vi "Initialise Hardware Splash 2.0.vi"(8 "error in (no error)":errorcluster) -> (0 "error out":errorcluster, 2 "VISA Refnum out":refnum<visa-resource-name>, 3 "Enabled Hardware out":T1={"Confocal"={"Enable"=TRUE, "Status"=FALSE, "Device"="Confocal"}, "Pinhole"={"Enable"=TRUE, "Status"=FALSE, "Device"="Pinhole"}, "PIFOC"={"Enable"=TRUE, "Status"=FALSE, "Device"="Piezo"}, "iFlex"={"Enable"=TRUE, "Status"=FALSE, "Device"="iFlex"}, "Manlight"={"Enable"=TRUE, "Status"=FALSE, "Device"="Manlight"}, "SLM"={"Enable"=TRUE, "Status"=FALSE, "Device"="SLM"}, "Camera"={"Enable"=FALSE, "Status"=FALSE, "Device"="Camera"}})   [LabVIEW 2020]
uses:
  _Controls/Enabled Hardware.ctl
panel:
  out "All Enabled and connected":bool
  in  "Enabled Hardware":T1={"Confocal"={"Enable"=TRUE, "Status"=FALSE, "Device"="Confocal"}, "Pinhole"={"Enable"=TRUE, "Status"=FALSE, "Device"="Pinhole"}, "PIFOC"={"Enable"=TRUE, "Status"=FALSE, "Device"="Piezo"}, "iFlex"={"Enable"=TRUE, "Status"=FALSE, "Device"="iFlex"}, "Manlight"={"Enable"=TRUE, "Status"=FALSE, "Device"="Manlight"}, "SLM"={"Enable"=TRUE, "Status"=FALSE, "Device"="SLM"}, "Camera"={"Enable"=FALSE, "Status"=FALSE, "Device"="Camera"}}
  in  "Review":bool
  in  "Scan For Missing":bool
  in  "animation":u16(ring)
  out "Status":string
  in  "Start":bool
  # "TweezerTron"
  # "Scanning for system hardware."
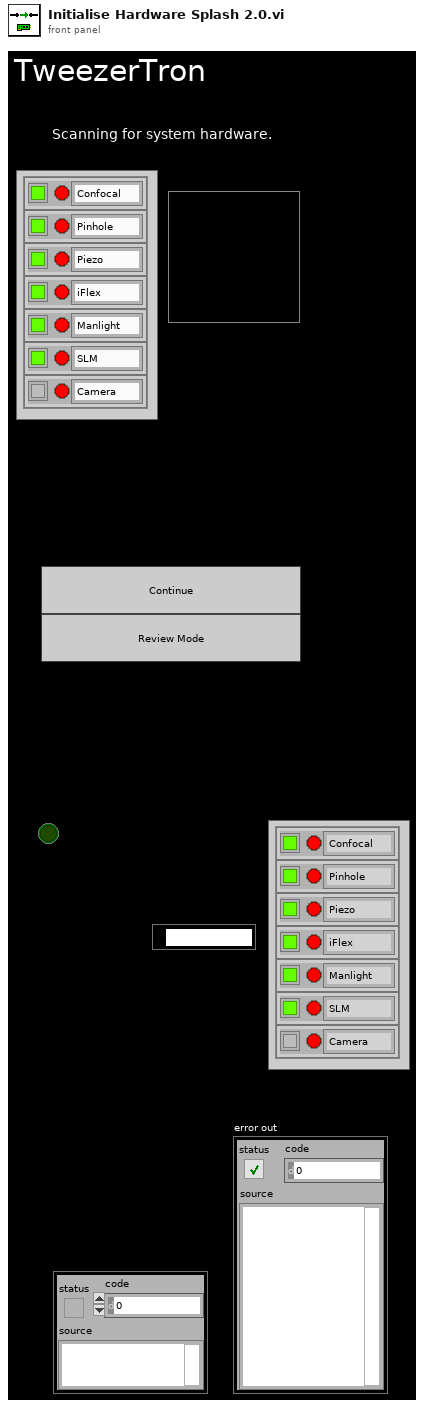
[diagram p1: front panel]
types:
  T1 = typedef "Enabled Hardware.ctl" = cluster{"Confocal":cluster{"Enable":bool, "Status":bool, "Device":string}, "Pinhole":cluster{"Enable":bool, "Status":bool, "Device":string}, "PIFOC":cluster{"Enable":bool, "Status":bool, "Device":string}, "iFlex":cluster{"Enable":bool, "Status":bool, "Device":string}, "Manlight":cluster{"Enable":bool, "Status":bool, "Device":string}, "SLM":cluster{"Enable":bool, "Status":bool, "Device":string}, "Camera":cluster{"Enable":bool, "Status":bool, "Device":string}}
  T2 = cluster{"Enable":bool, "Status":bool, "Device":string}
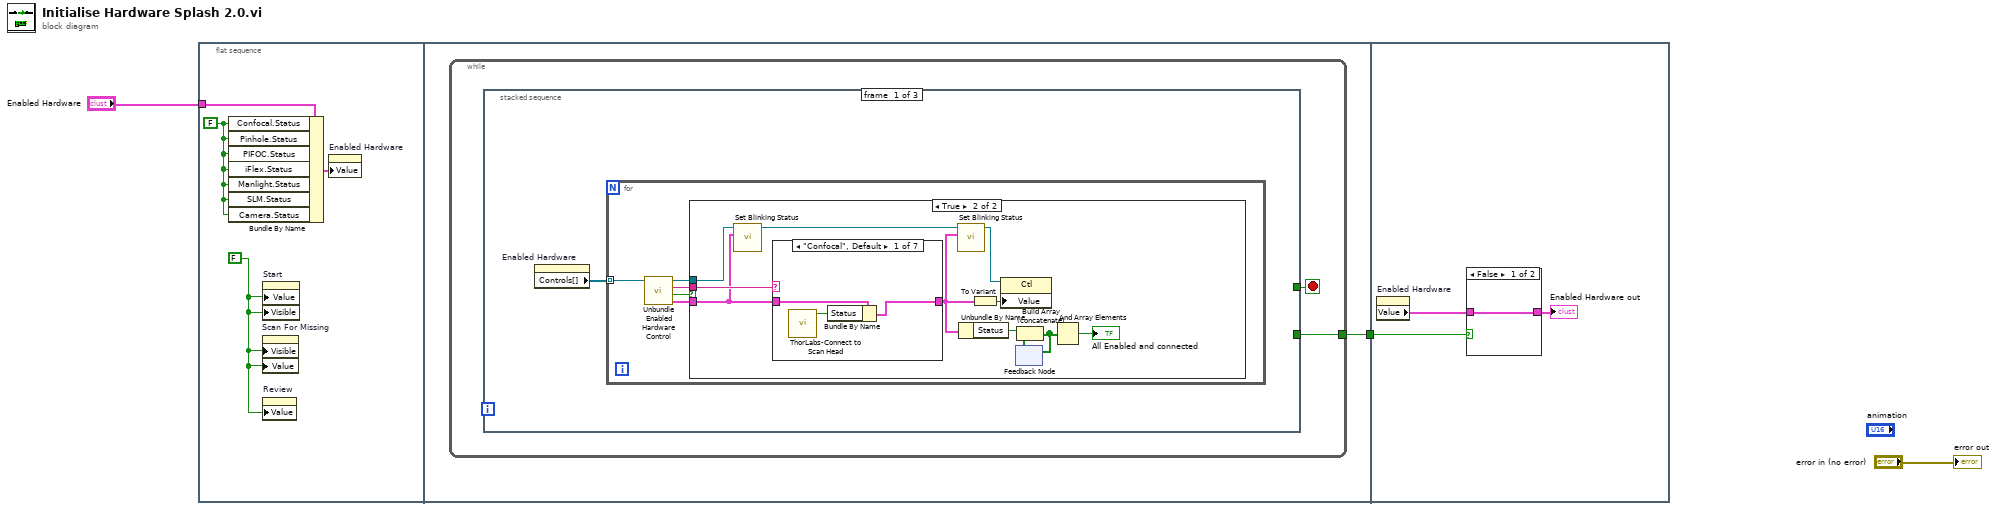
[diagram p0: block diagram]
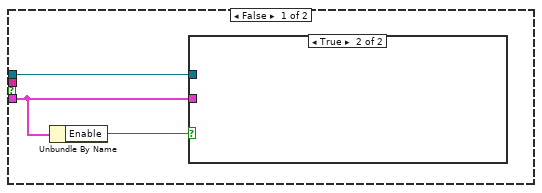
[diagram p2: hidden frame]
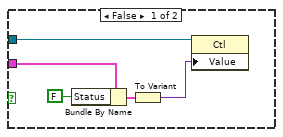
[diagram p3: hidden frame]
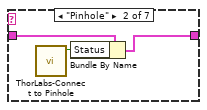
[diagram p4: hidden frame]
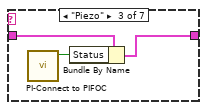
[diagram p5: hidden frame]
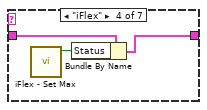
[diagram p6: hidden frame]
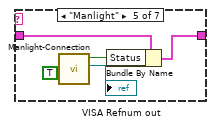
[diagram p7: hidden frame]
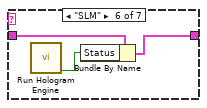
[diagram p8: hidden frame]
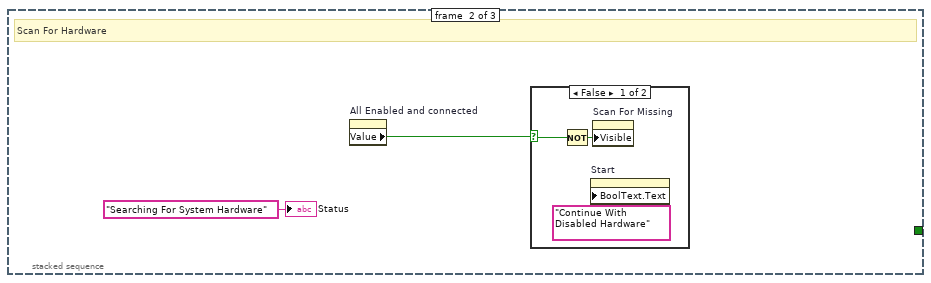
[diagram p10: hidden frame]
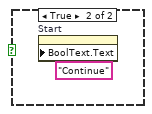
[diagram p11: hidden frame]
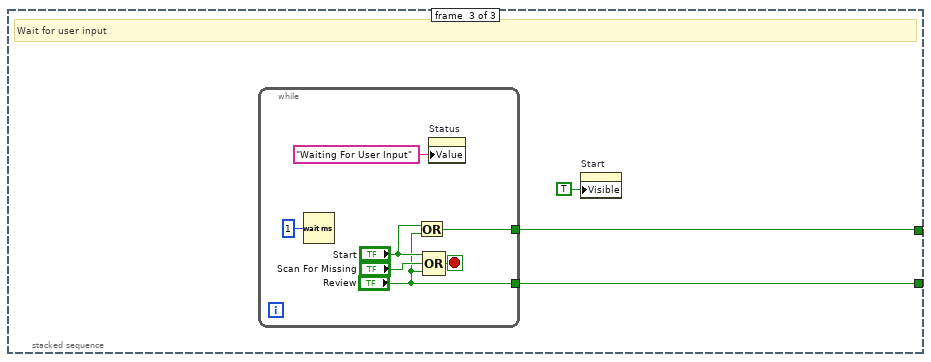
[diagram p12: hidden frame]
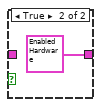
[diagram p13: hidden frame]
diagram:
  n1 = flat-sequence {
    tunnel: "Enabled Hardware" -> [w6]
    tunnel: [w8] -> w1
    tunnel: w1 -> [w73]
    frame #0 {
      w5 = FALSE ("Confocal")
      w7 = FALSE ("Confocal")
      n2 = Bundle By Name(cluster=w6, "Confocal.Status"=w5, "Pinhole.Status"=w5, "PIFOC.Status"=w5, "iFlex.Status"=w5, "Manlight.Status"=w5, "SLM.Status"=w5, "Camera.Status"=w5) -> (w4:T1)
      n3 = property on="Scan For Missing" class="Bool"("Visible"=w7, "Value"=w7) -> ()  [unwired: 2 in, 2 out]
      n4 = property on="Start" class="Bool (strict)"("Value"=w7, "Visible"=w7) -> ()  [unwired: 2 in, 2 out]
      n5 = property on="Review" class="Bool (strict)"("Value"=w7) -> ()  [unwired: 2 in, 2 out]
      n6 = property on="Enabled Hardware" class="Clust (strict)"("Value"=w4) -> ()  [unwired: 2 in, 2 out]
    }
    frame #1 {
      n7 = while {
        tunnel: [w10] -> w8
        stop <- w9 stop-if-true
        n8 = stacked-sequence {
          tunnel: [_ _ w65] -> w9
          tunnel: [_ _ w64] -> w10
          frame #0 {
            n9 = property on="Enabled Hardware" class="Clust (strict)"() -> ("Controls[]"=w11:refnum<vi>[])  [unwired: 2 in, 2 out]
            n10 = for {
              tunnel: w11 -> [w14] mode=indexing
              n11 = call "Unbundle Enabled Hardware Control.vi"("Control in"=w14) -> ("data out"=w15:T2, "Enabled and not yet connected"=w12:bool, "Device"=w16:string, "Control out"=w13:refnum<vi>)  [unwired: 7 in]
              n12 = case shown="True" w12 {
                tunnel: w16 -> [_ w35]
                tunnel: w15 -> [w18 w31]
                tunnel: w13 -> [w19 w32]
                frame False {
                  n13 = Unbundle By Name(w18) -> ("Enable"=w17:bool)
                  n14 = case shown="True" w17 {
                    tunnel: w19 -> [w24 _]
                    tunnel: w18 -> [w20 _]
                    frame False {
                      n15 = Bundle By Name(cluster=w20, "Status"=FALSE) -> (w21:T2)
                      n16 = To Variant(anything=w21) -> (Variant=w22:variant)
                      n17 = property class="Ctl"(reference=w24, "Value"=w22) -> ()  [unwired: 1 in, 2 out]
                    }
                    frame True {
                    }
                  }
                }
                frame True {
                  n18 = call "Set Blinking Status.vi"("data in"=w31, "Control in"=w32) -> ("Control out"=w30:refnum<vi>)  [unwired: 9 in]
                  n19 = case shown="\"Confocal\", Default" w35 {
                    tunnel: w31 -> [w38 w41 w44 w47 w51 w55 w56]
                    tunnel: [w36 w40 w42 w45 w49 w53 w56] -> w28
                    frame "Confocal", Default {
                      n20 = call "ThorLabs-Connect to Scan Head.vi"() -> ("ThorLabs Scan Head Connected"=w37:bool)  [unwired: 10 in, 1 out]
                      n21 = Bundle By Name(cluster=w38, "Status"=w37) -> (w36:T2)
                    }
                    frame "Pinhole" {
                      n22 = call "ThorLabs-Connect to Pinhole.vi"() -> ("Thorlabs Pinhole Connected"=w39:bool)  [unwired: 10 in, 1 out]
                      n23 = Bundle By Name(cluster=w41, "Status"=w39) -> (w40:T2)
                    }
                    frame "Piezo" {
                      n24 = call "PI-Connect to PIFOC.vi"() -> ("No Errors"=w43:bool)  [unwired: 5 in, 2 out]
                      n25 = Bundle By Name(cluster=w44, "Status"=w43) -> (w42:T2)
                    }
                    frame "iFlex" {
                      n26 = call "iFlex - Set Max.vi"() -> ("iFlex Enabled"=w46:bool)  [unwired: 11 in]
                      n27 = Bundle By Name(cluster=w47, "Status"=w46) -> (w45:T2)
                    }
                    frame "Manlight" {
                      n28 = call "Manlight-Connection.vi"("Connect?"=TRUE ("Connect")) -> ("VISA Refnum out"=→"VISA Refnum out":refnum<visa-resource-name>, "Manlight Laser Connected"=w50:bool)  [unwired: 3 in, 2 out]
                      n29 = Bundle By Name(cluster=w51, "Status"=w50) -> (w49:T2)
                    }
                    frame "SLM" {
                      n30 = call "Run Hologram Engine.vi"() -> ("status"=w54:bool)  [unwired: 11 in]
                      n31 = Bundle By Name(cluster=w55, "Status"=w54) -> (w53:T2)
                    }
                    frame "Camera" {
                    }
                  }
                  n32 = call "Set Blinking Status.vi"("data in"=w28, "Control in"=w30) -> ("Control out"=w33:refnum<vi>)  [unwired: 9 in]
                  n33 = Unbundle By Name(w28) -> ("Status"=w27:bool)
                  n34 = To Variant(anything=w28) -> (Variant=w34:variant)
                  n35 = property class="Ctl"(reference=w33, "Value"=w34) -> ()  [unwired: 1 in, 2 out]
                  n36 = feedback #1() -> (w29:bool[])  [unwired: 1 in]
                  n37 = Build Array (concatenate)(w27, w29) -> (w26:bool[])
                  n38 = feedback-in #1(w26) -> ()
                  n39 = And Array Elements(Boolean array=w26) -> (logical AND=→"All Enabled and connected":bool)
                }
              }
            }
          }
          frame #1 {
            # "Scan For Hardware"
            n40 = property on="All Enabled and connected" class="Bool (strict)"() -> ("Value"=w57:bool)  [unwired: 2 in, 2 out]
            n41 = case shown="False" w57 {
              selector: w57 -> [w60 _]
              frame False {
                n42 = Not(x=w60) -> (.not. x?=w59:bool)
                n43 = property on="Start" class="Bool (strict)"("BoolText.Text"="Continue With Disabled Hardware") -> ()  [unwired: 2 in, 2 out]
                n44 = property on="Scan For Missing" class="Bool"("Visible"=w59) -> ()  [unwired: 2 in, 2 out]
              }
              frame True {
                n45 = property on="Start" class="Bool (strict)"("BoolText.Text"="Continue" ("Boolean Text.Text")) -> ()  [unwired: 2 in, 2 out]
              }
            }
            "Status" <- "Searching For System Hardware" ("string")
          }
          frame #2 {
            # "Wait for user input"
            n46 = while {
              tunnel: [w68] -> w65
              tunnel: ["Review"] -> w64
              stop <- w70 stop-if-true
              n47 = Wait (ms)(milliseconds to wait=u32 1) -> ()  [unwired: 1 out]
              n48 = Or(x="Start", y="Review") -> (x .or. y?=w68:bool)
              n49 = Compound Arithmetic op=OR("Start", "Scan For Missing", "Review") -> (w70:bool)
              n50 = property on="Status" class="Str"("Value"="Waiting For User Input" ("Status")) -> ()  [unwired: 2 in, 2 out]
            }
            n51 = property on="Start" class="Bool (strict)"("Visible"=TRUE) -> ()  [unwired: 2 in, 2 out]
          }
        }
      }
    }
    frame #2 {
      n52 = property on="Enabled Hardware" class="Clust (strict)"() -> ("Value"=w75:T1)  [unwired: 2 in, 2 out]
      n53 = case shown="False" w73 {
        tunnel: [w76 T1 {"Confocal"={"Enable"=FALSE, "Status"=FALSE, "Device"="Confocal"}, "Pinhole"={"Enable"=FALSE, "Status"=FALSE, "Device"="Pinhole"}, "PIFOC"={"Enable"=FALSE, "Status"=FALSE, "Device"="Piezo"}, "iFlex"={"Enable"=FALSE, "Status"=FALSE, "Device"="iFlex"}, "Manlight"={"Enable"=FALSE, "Status"=FALSE, "Device"="Manlight"}, "SLM"={"Enable"=FALSE, "Status"=FALSE, "Device"="SLM"}, "Camera"={"Enable"=FALSE, "Status"=FALSE, "Device"="Camera"}} ("Enabled Hardware")] -> w74
        tunnel: w75 -> [w76 _]
        frame False {
        }
        frame True {
        }
      }
      "Enabled Hardware out" <- w74
    }
  }
  "error out" <- "error in (no error)"
